vi "TC_AppendToRefArray.vi"(4 "name":string, 5 "arrayIn":T1, 6 "ref6":refnum<vi>, 7 "ref1":refnum<vi>, 8 "ref5":refnum<vi>, 9 "ref4":refnum<vi>, 10 "ref3":refnum<vi>, 11 "ref2":refnum<vi>) -> (0 "arrayOut":T1)   [LabVIEW 2017]
uses:
  RefArray.ctl
panel:
  in  "ref6 2":refnum<vi>
  in  "ref3 2":refnum<vi>
  in  "ref4 2":refnum<vi>
  in  "ref5 2":refnum<vi>
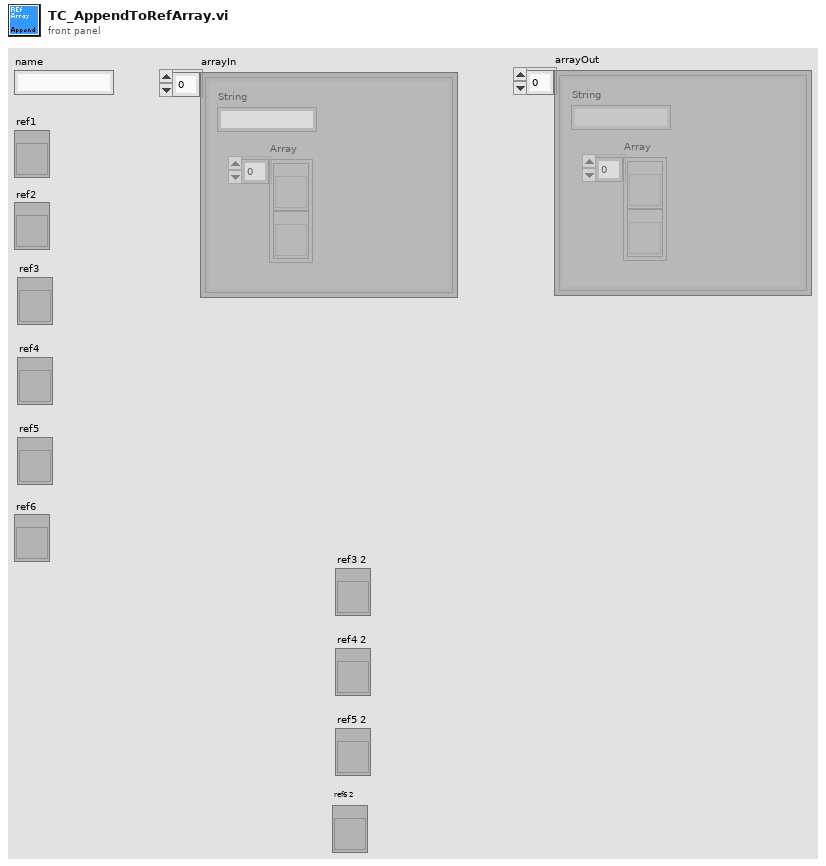
[diagram p1: front panel]
types:
  T1 = typedef "RefArray.ctl" = cluster{"String":string, "Array":refnum<vi>[]}[]
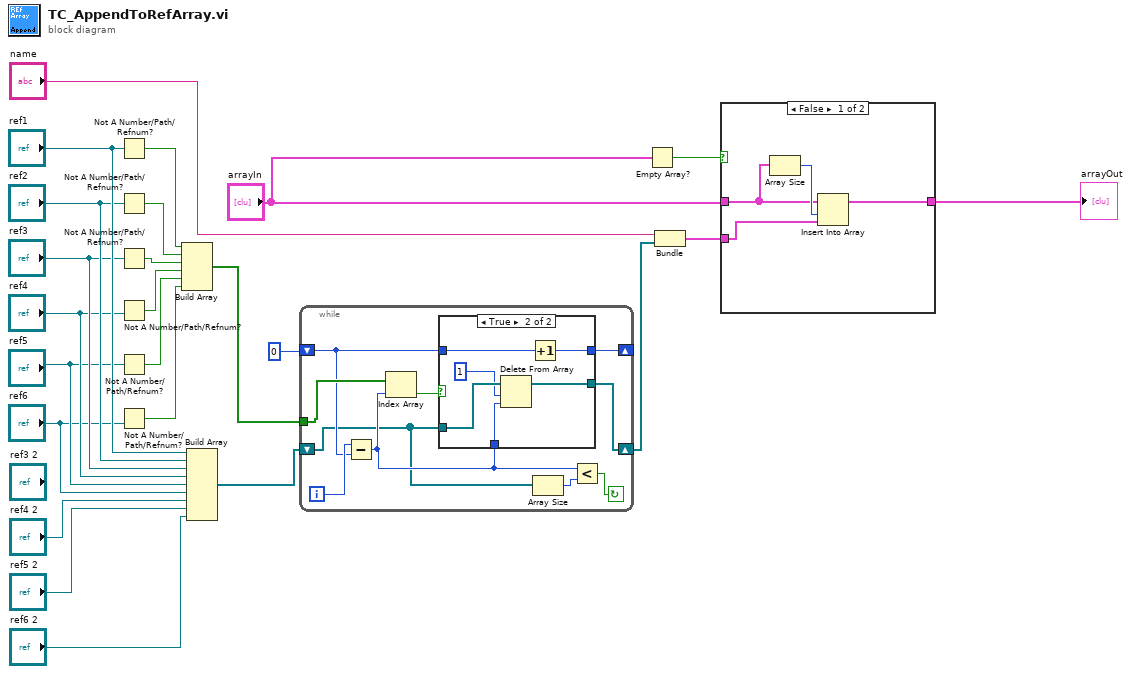
[diagram p0: block diagram]
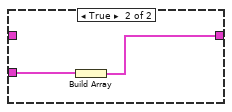
[diagram p2: hidden frame]
diagram:
  n1 = Not A Number/Path/Refnum?(number/path/refnum="ref1") -> (NaN/Path/Refnum?=w24:bool)
  n2 = Not A Number/Path/Refnum?(number/path/refnum="ref2") -> (NaN/Path/Refnum?=w23:bool)
  n3 = Not A Number/Path/Refnum?(number/path/refnum="ref3") -> (NaN/Path/Refnum?=w22:bool)
  n4 = Not A Number/Path/Refnum?(number/path/refnum="ref4") -> (NaN/Path/Refnum?=w21:bool)
  n5 = Not A Number/Path/Refnum?(number/path/refnum="ref5") -> (NaN/Path/Refnum?=w19:bool)
  n6 = Not A Number/Path/Refnum?(number/path/refnum="ref6") -> (NaN/Path/Refnum?=w20:bool)
  n7 = Build Array(w24, w23, w22, w21, w19, w20) -> (w10:bool[])
  n8 = Build Array("ref1", "ref2", "ref3", "ref4", "ref5", "ref6", "ref4 2", "ref5 2", "ref6 2") -> (w11:refnum<vi>[])
  n9 = while {
    tunnel: w10 -> [w32]
    shift-right: [w30] -> w9
    shift-left: w11 -> [w25]
    shift-right: [w29] -> _
    shift-left: 0 -> [w27]
    i -> [w28]
    stop <- w33 continue-if-true
    n10 = Subtract(x=w28, y=w27) -> (x-y=w26:i32)
    n11 = Index Array(array=w32, index=w26) -> (element=w31:bool)
    n12 = case shown="True" w31 {
      tunnel: w25 -> [w36 w42]
      tunnel: [w36 w40] -> w30
      tunnel: w27 -> [w35 w39]
      tunnel: [w35 w38] -> w29
      tunnel: w26 -> [_ w37]
      frame False {
      }
      frame True {
        n13 = Delete From Array(array=w42, length=1, index=w37) -> (array with subset deleted=w40:refnum<vi>[])  [unwired: 1 out]
        n14 = Increment(x=w39) -> (x+1=w38:i32)
      }
    }
    n15 = Array Size(array=w25) -> (size(s)=w34:i32)
    n16 = Less?(x=w26, y=w34) -> (x < y?=w33:bool)
  }
  n17 = Empty Array?(array="arrayIn") -> (empty?=w7:bool)
  n18 = Bundle("name"="name", w9) -> (w5:cluster{"name":string, refnum<vi>[]})  [unwired: 1 in]
  n19 = case shown="False" w7 {
    tunnel: "arrayIn" -> [w45 _]
    tunnel: w5 -> [w44 w48]
    tunnel: [w43 w47] -> w4
    frame False {
      n20 = Array Size(array=w45) -> (size(s)=w46:i32)
      n21 = Insert Into Array(array=w45, index=w46, new element=w44) -> (w43:T1)
    }
    frame True {
      n22 = Build Array(w48) -> (w47:cluster{"name":string, refnum<vi>[]}[])
    }
  }
  "arrayOut" <- w4
